vi "Read Valid Messages.vi"(8 "error in (no error)":errorcluster, 11 "Pump Controller in":refnum<class "Pump Controller.lvclass">) -> (0 "error out":errorcluster, 2 "Valid Messages":string[](array[string]), 3 "Pump Controller out":refnum<class "Pump Controller.lvclass">)   [LabVIEW 2020, in "Pump Controller.lvclass"]
uses:
  Pump Controller.lvclass
  Pump Controller.lvclass/Pump Controller.ctl
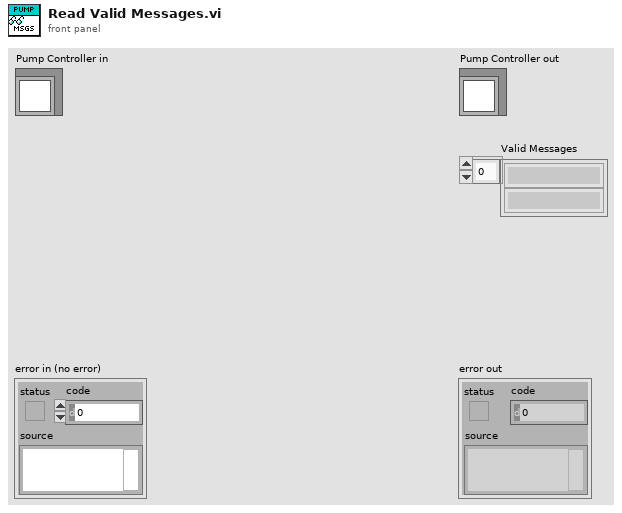
[diagram p1: front panel]
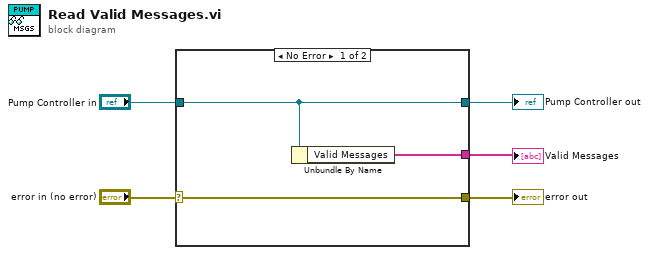
[diagram p0: block diagram]
diagram:
  n1 = case shown="No Error" "error in (no error)" {
    selector: "error in (no error)" -> [w6 w10]
    tunnel: "Pump Controller in" -> [w7 w9]
    tunnel: [w8 _] -> w3
    tunnel: [w7 w9] -> w4
    tunnel: [w6 w10] -> w2
    frame No Error {
      n2 = Unbundle By Name(w7) -> ("Valid Messages"=w8:string[])
    }
    frame Error {
    }
  }
  "error out" <- w2
  "Pump Controller out" <- w4
  "Valid Messages" <- w3
